vi "AND_Filter.vi"(8 "Error out":errorcluster, 9 "Show Hierarhy":T1={"Show hierarhy in first column(F)"=FALSE, "Left separator"="[", "Right separator"="] "}, 10 "Matches Filter [AND]":cluster{"Matches String":string, "Column":i32}[](array[cluster]), 11 "Tree in":refnum<class "Tree.lvclass">) -> (0 "Error out":errorcluster, 3 "Tree out":refnum<class "Tree.lvclass">)   [LabVIEW 2021, in "Tree.lvlib" / "Tree.lvclass"]
uses:
  Tree.lvclass
  Private/TreeControllerTag.ctl
  Tree.lvclass/Tree.ctl
panel:
  # "Use (Column = -1) to search coincidence in any column"
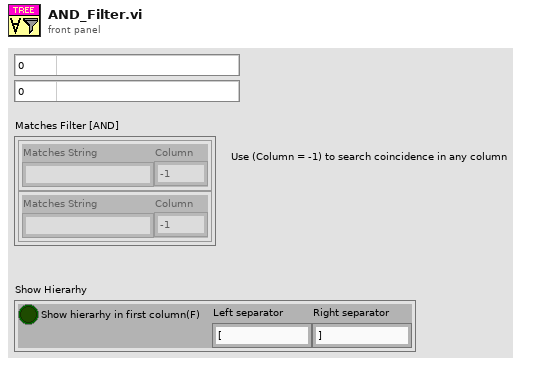
[diagram p1: front panel]
types:
  T1 = cluster{"Show hierarhy in first column(F)":bool, "Left separator":string, "Right separator":string}
  T2 = typedef "Tree.lvlib/Tree.lvclass/TreeControllerTag.ctl" = enum8{"Null", "1. Add item", "2. Delete item", "3. Get All Tree Data", "4. Drag Starting", "5. Drag Ended", "6. Add Tree Values", "7. Get Item Value", "8. Edit Item", "9. StepBack", "10. Filter"}
  T3 = cluster{enum8{"AND", "OR", "NOT AND", "NOT OR"}, "Matches Filter [AND]":cluster{"Matches String":string, "Column":i32}[], "Show Hierarhy":cluster{"Show hierarhy in first column(F)":bool, "Left separator":string, "Right separator":string}}
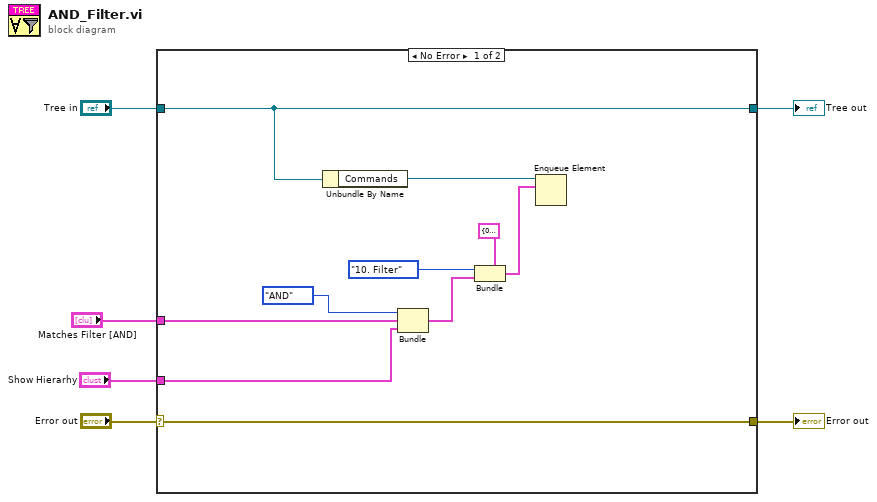
[diagram p0: block diagram]
diagram:
  n1 = case shown="No Error" "Error out" {
    selector: "Error out" -> [w16 w18]
    tunnel: [w16 w18] -> w5
    tunnel: [w14 w17] -> w3
    tunnel: "Tree in" -> [w14 w17]
    tunnel: "Show Hierarhy" -> [w9 _]
    tunnel: "Matches Filter [AND]" -> [w8 _]
    frame No Error {
      n2 = Unbundle By Name(w14) -> ("Commands"=w15:refnum<queue>)
      n3 = Bundle(enum8{"AND", "OR", "NOT AND", "NOT OR"}."AND", "Matches Filter [AND]"=w8, "Show Hierarhy"=w9) -> (w10:T3)  [unwired: 1 in]
      n4 = Bundle(cluster=cluster{"Tag":u8, "Value":variant} {"Tag"=0, "Value"=variant} ("element"), "Tag"=TreeControllerTag."10. Filter", "Value"=w10) -> (w12:cluster{"Tag":u8, "Value":variant})
      n5 = Enqueue Element(queue=w15, element=w12) -> ()  [unwired: 2 in, 3 out]
    }
    frame Error {
    }
  }
  "Error out" <- w5
  "Tree out" <- w3
